vi "sv_Calculate Band Power.vi"(1 "octave info":T1={"standard"=enum."ANSI S1.11", "bandwidth"=enum."1 octave", "low band"=0, "high band"=0, "weighting filter"=0, "dB reference"=0.0, "dB On"=FALSE, "unit label"="", "channel name"="", "description"="", "engineering units"=1, "custom label"="", "spectrum type"=enum."magnitude", "spectral density"=FALSE, "filters settled"=FALSE} {"engineering units" items=["custom..."=0, "V"=1, "A"=21, "C"=30, "pC"=31, "s"=32, "-"=29, "Pa"=2, "N"=20, "g"=3, "m/s^2"=4, "m/s"=5, "m"=6, "mm/s"=12, "mm"=13, "micron/s"=14, "micron"=15, "in/s^2"=7, "in/s"=8, "in"=9, "mil/s"=10, "mil"=11, "rad/s^2"=16, "rad/s"=17, "rad"=18, "deg/s^2"=26, "deg/s"=27, "deg"=28, "RPM"=22, "cycle/s^2"=23, "Hz"=24, "cycle"=25, "strain"=19]; "dB reference" format="%.2e"; "weighting filter" items=["Linear", "A-weighting", "B-weighting", "C-weighting", "ITU-R 468-4", "Dolby", "CCITT", "C-message", "Wb", "Wc", "Wd", "We", "Wf", "Wh", "Wj", "Wk", "Wm", "AES17 20 kHz lowpass", "AES17 40 kHz lowpass", "AES17 20 kHz highpass", "AES17 40 kHz highpass"]}, 2 "octave spectrum":T5 {"band power [dB EU]" format="%.2f"; "nominal frequencies [Hz]" format="%.2f"}) -> (0 "total band power":dbl)   [LabVIEW 2017, in "SoundVib_Octave.lvlib"]
doc: "This VI calculates the <B>total band power [dB EU]</B> of the <B>octave spectrum</B>"
uses:
  <vilib>/addons/Sound and Vibration/svt_Octave/SoundVib_Octave.lvlib
  <vilib>/addons/_NISVFA/_Shared subVIs/Controls/svc_Octave Info.ctl
  <vilib>/addons/_NISVFA/_Shared subVIs/Controls/svc_Octave Standard.ctl
  <vilib>/addons/_NISVFA/_Shared subVIs/Controls/svc_Weighting Filter Text Ring.ctl
  <vilib>/addons/_NISVFA/_Shared subVIs/Controls/svc_Engineering Units Text Ring.ctl
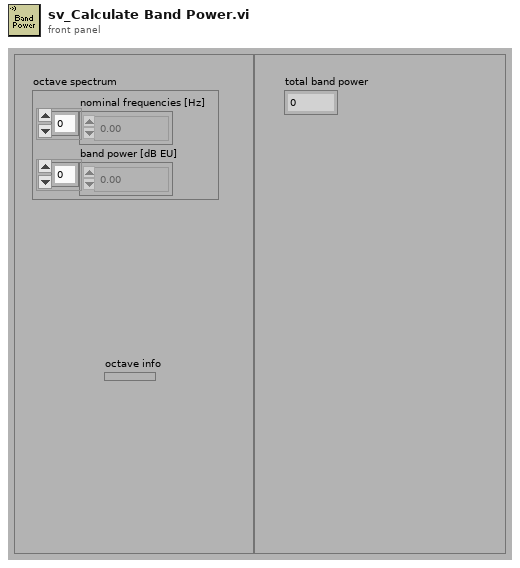
[diagram p1: front panel]
types:
  T1 = typedef "svc_Octave Info.ctl" = cluster{"standard":T2, "bandwidth":enum16{"1 octave", "1/3 octave", "1/6 octave", "1/12 octave", "1/24 octave"}, "low band":i32, "high band":i32, "weighting filter":T3, "dB reference":dbl, "dB On":bool, "unit label":string, "channel name":string, "description":string, "engineering units":T4, "custom label":string, "spectrum type":enum16{"power", "magnitude"}, "spectral density":bool, "filters settled":bool}
  T2 = typedef "svc_Octave Standard.ctl" = enum16{"ANSI S1.11", "IEC 61260"}
  T3 = typedef "svc_Weighting Filter Text Ring.ctl" = u16
  T4 = typedef "svc_Engineering Units Text Ring.ctl" = u16
  T5 = cluster{"nominal frequencies [Hz]":dbl[], "band power [dB EU]":dbl[]}
  T6 = enum16{"1 octave", "1/3 octave", "1/6 octave", "1/12 octave", "1/24 octave"}
  T7 = enum16{"1 octave", "1/3 octave", "1/6 octave", "1/12 octave", "1/24 octave", "1/48 octave", "1/96 octave"}
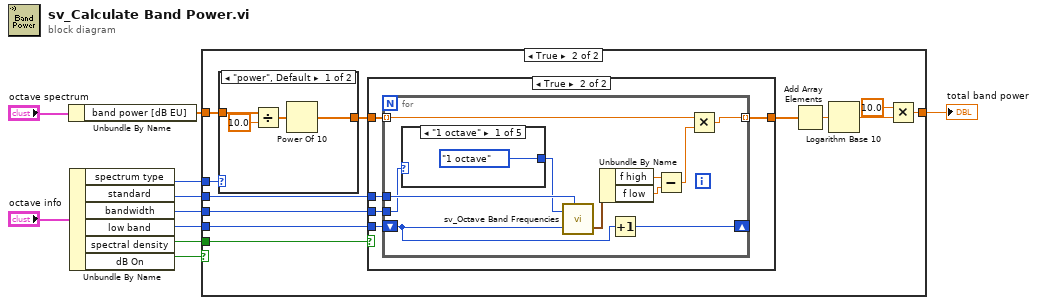
[diagram p0: block diagram]
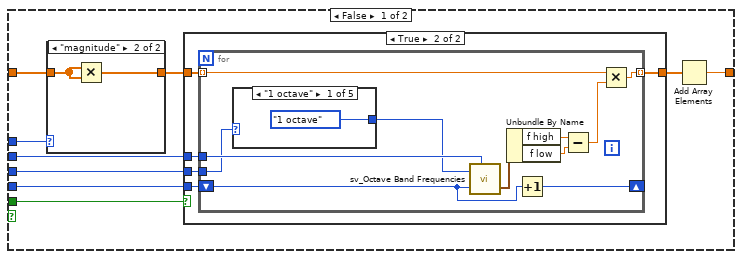
[diagram p2: hidden frame]
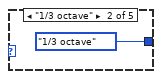
[diagram p4: hidden frame]
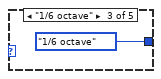
[diagram p5: hidden frame]
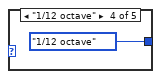
[diagram p6: hidden frame]
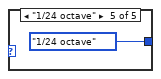
[diagram p7: hidden frame]
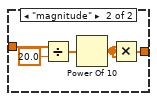
[diagram p9: hidden frame]
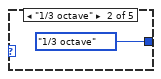
[diagram p11: hidden frame]
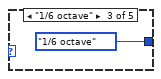
[diagram p12: hidden frame]
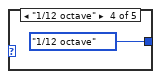
[diagram p13: hidden frame]
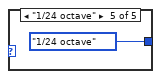
[diagram p14: hidden frame]
diagram:
  n1 = Unbundle By Name("octave spectrum") -> ("band power [dB EU]"=w3:dbl[])
  n2 = Unbundle By Name("octave info") -> ("spectrum type"=w2:enum16{"power", "magnitude"}, "standard"=w6:T2, "bandwidth"=w5:T6, "low band"=w7:i32, "spectral density"=w1:bool, "dB On"=w9:bool)
  n3 = case shown="True" w9 {
    tunnel: [w19 w54] -> w8
    tunnel: w7 -> [w18 w49]
    tunnel: w6 -> [w17 w47]
    tunnel: w5 -> [w16 w48]
    tunnel: w3 -> [w13 w53]
    tunnel: w2 -> [w14 w46]
    tunnel: w1 -> [w11 w50]
    frame False {
      n4 = case shown="\"magnitude\"" w14 {
        tunnel: w13 -> [w42 w44]
        tunnel: [w42 w43] -> w12
        frame "power", Default {
        }
        frame "magnitude" {
          n5 = Multiply(x=w44, y=w44) -> (x*y=w43:dbl[])
        }
      }
      n6 = case shown="True" w11 {
        tunnel: w18 -> [_ w25]
        tunnel: w17 -> [_ w24]
        tunnel: w16 -> [_ w23]
        tunnel: [w20 w22] -> w15
        tunnel: w12 -> [w20 w21]
        frame False {
        }
        frame True {
          n7 = for {
            tunnel: w21 -> [w29] mode=indexing
            shift-right: [w36] -> _
            shift-left: w25 -> [w34]
            tunnel: w24 -> [w35]
            tunnel: w23 -> [w27]
            tunnel: [w28] -> w22 mode=indexing
            n8 = case shown="\"1 octave\"" w27 {
              tunnel: [T7."1 octave" ("bandwidth") T7."1/3 octave" ("bandwidth") T7."1/6 octave" ("bandwidth") T7."1/12 octave" ("bandwidth") T7."1/24 octave" ("bandwidth")] -> w26
              frame "1 octave" {
              }
              frame "1/3 octave" {
              }
              frame "1/6 octave" {
              }
              frame "1/12 octave" {
              }
              frame "1/24 octave" {
              }
            }
            n9 = call <vilib>:"sv_Octave Band Frequencies.vi"("octave band selector"=w34, "bandwidth"=w26, "standard"=w35) -> ("bandedge frequencies [Hz]"=w33:cluster{"f low":dbl, "f high":dbl})  [unwired: 1 in, 3 out]
            n10 = Unbundle By Name(w33) -> ("f high"=w32:dbl, "f low"=w31:dbl)
            n11 = Increment(x=w34) -> (x+1=w36:i32)
            n12 = Subtract(x=w32, y=w31) -> (x-y=w30:dbl)
            n13 = Multiply(x=w29, y=w30) -> (x*y=w28:dbl)
          }
        }
      }
      n14 = Add Array Elements(numeric array=w15) -> (sum=w19:dbl)
    }
    frame True {
      n15 = case shown="\"power\", Default" w46 {
        tunnel: w53 -> [w60 w65]
        tunnel: [w58 w63] -> w52
        frame "power", Default {
          n16 = Divide(x=w60, y=10.0) -> (x/y=w57:dbl[])
          n17 = Power Of 10(x=w57) -> (10^x=w58:dbl[])
        }
        frame "magnitude" {
          n18 = Divide(x=w65, y=20.0) -> (x/y=w64:dbl[])
          n19 = Power Of 10(x=w64) -> (10^x=w62:dbl[])
          n20 = Multiply(x=w62, y=w62) -> (x*y=w63:dbl[])
        }
      }
      n21 = case shown="True" w50 {
        tunnel: w49 -> [_ w71]
        tunnel: w47 -> [_ w70]
        tunnel: w48 -> [_ w69]
        tunnel: [w66 w68] -> w51
        tunnel: w52 -> [w66 w67]
        frame False {
        }
        frame True {
          n22 = for {
            tunnel: w67 -> [w75] mode=indexing
            shift-right: [w82] -> _
            shift-left: w71 -> [w80]
            tunnel: w70 -> [w81]
            tunnel: w69 -> [w72]
            tunnel: [w74] -> w68 mode=indexing
            n23 = case shown="\"1 octave\"" w72 {
              tunnel: [T7."1 octave" ("bandwidth") T7."1/3 octave" ("bandwidth") T7."1/6 octave" ("bandwidth") T7."1/12 octave" ("bandwidth") T7."1/24 octave" ("bandwidth")] -> w73
              frame "1 octave" {
              }
              frame "1/3 octave" {
              }
              frame "1/6 octave" {
              }
              frame "1/12 octave" {
              }
              frame "1/24 octave" {
              }
            }
            n24 = call <vilib>:"sv_Octave Band Frequencies.vi"("octave band selector"=w80, "bandwidth"=w73, "standard"=w81) -> ("bandedge frequencies [Hz]"=w79:cluster{"f low":dbl, "f high":dbl})  [unwired: 1 in, 3 out]
            n25 = Unbundle By Name(w79) -> ("f high"=w78:dbl, "f low"=w77:dbl)
            n26 = Increment(x=w80) -> (x+1=w82:i32)
            n27 = Subtract(x=w78, y=w77) -> (x-y=w76:dbl)
            n28 = Multiply(x=w75, y=w76) -> (x*y=w74:dbl)
          }
        }
      }
      n29 = Add Array Elements(numeric array=w51) -> (sum=w56:dbl)
      n30 = Logarithm Base 10(1:w56) -> (0:w55:dbl)
      n31 = Multiply(x=10.0 ("y"), y=w55) -> (x*y=w54:dbl)
    }
  }
  "total band power" <- w8
